vi "Hg-system-wendy.vi"() -> ()   [LabVIEW 2015]
uses:
  labview_Hg/XPALTC V 1.0 Andrey/Devices/Sirah Control 3 (provided by Sirah)/Addon/LabVIEW - Grobi API/Source/Laser/SC API Unit.ctl
panel:
  in  "VISA resource -Energy Meter 2":refnum<visa-resource-name>
  out "Current Pulse Energy Value 2":dbl=5.0 caption="Value"
  out "Current Pulse Energy Value Chart 2":dbl(graph)
  in  "VISA resource -Energy Meter":refnum<visa-resource-name>
  out "Current Pulse Energy Value":dbl=5.0 caption="Value"
  out "Current Pulse Energy Value Chart":dbl(graph)
  out "Current loop #":dbl format="%.4f"
  in  "# of Waveforms":i32
  in  "stop for waveform loop":bool
  out "Waveform Graph":dbl[](graph)
  in  "Channel":i32
  in  "VISA resource - Oscilliscope":refnum<visa-resource-name>
  out "Current Wavelength Read (nm)":dbl format="%.4f"
  out "Current Wavelength  Minus (nm)":dbl format="%.4f"
  in  "Boolean":bool
  out "Begin Wavelength Read (nm)":dbl format="%.4f"
  out "Begin Wavelength Read after laser go to (nm)":dbl format="%.4f"
  in  "Scan Step, nm":dbl
  in  "Scan to(longer), nm":dbl
  in  "Scan from (shorter), nm":dbl
  in  "VISA Resource - Dye Laser":refnum<visa-resource-name>
  out "error out":errorcluster
  in  "error in (no error)":errorcluster
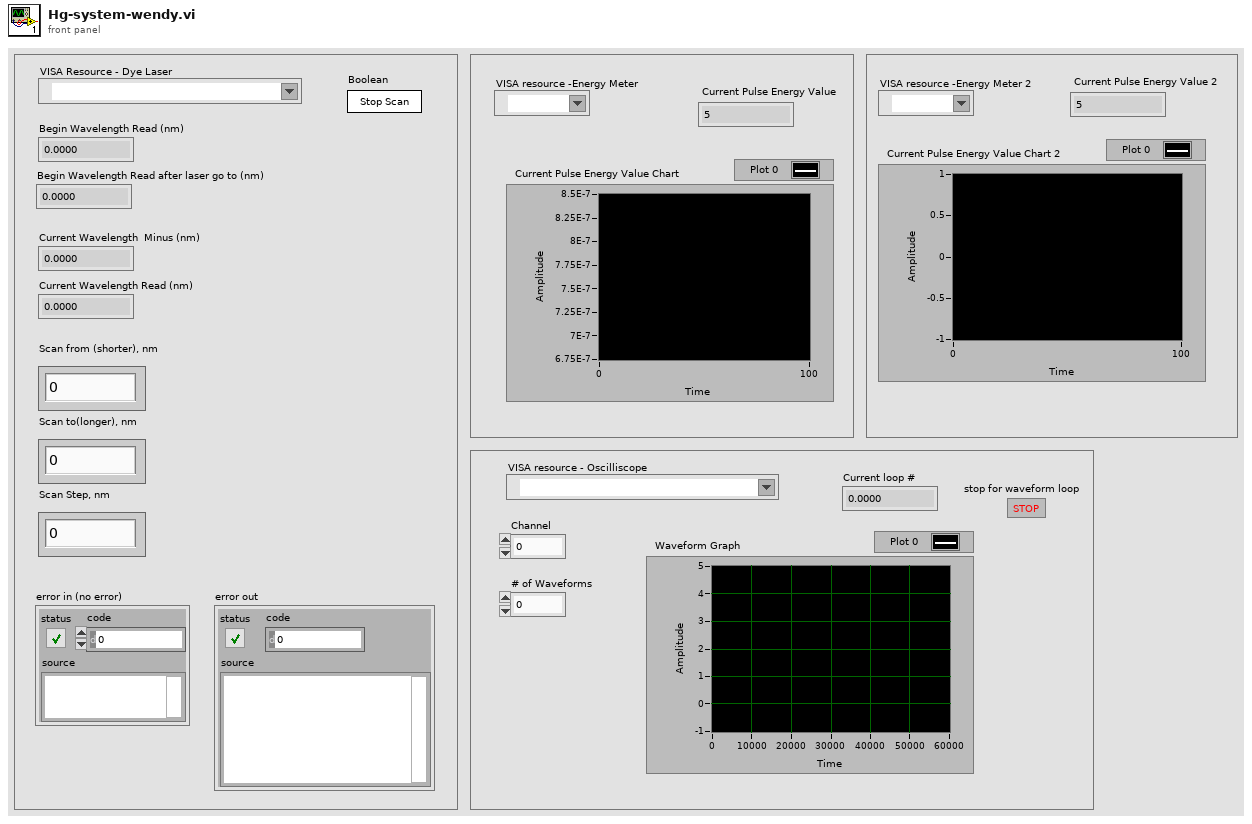
[diagram p1: front panel]
types:
  T1 = typedef "SC API Unit.ctl" = enum16{"nm", "THz", "1/cm"}
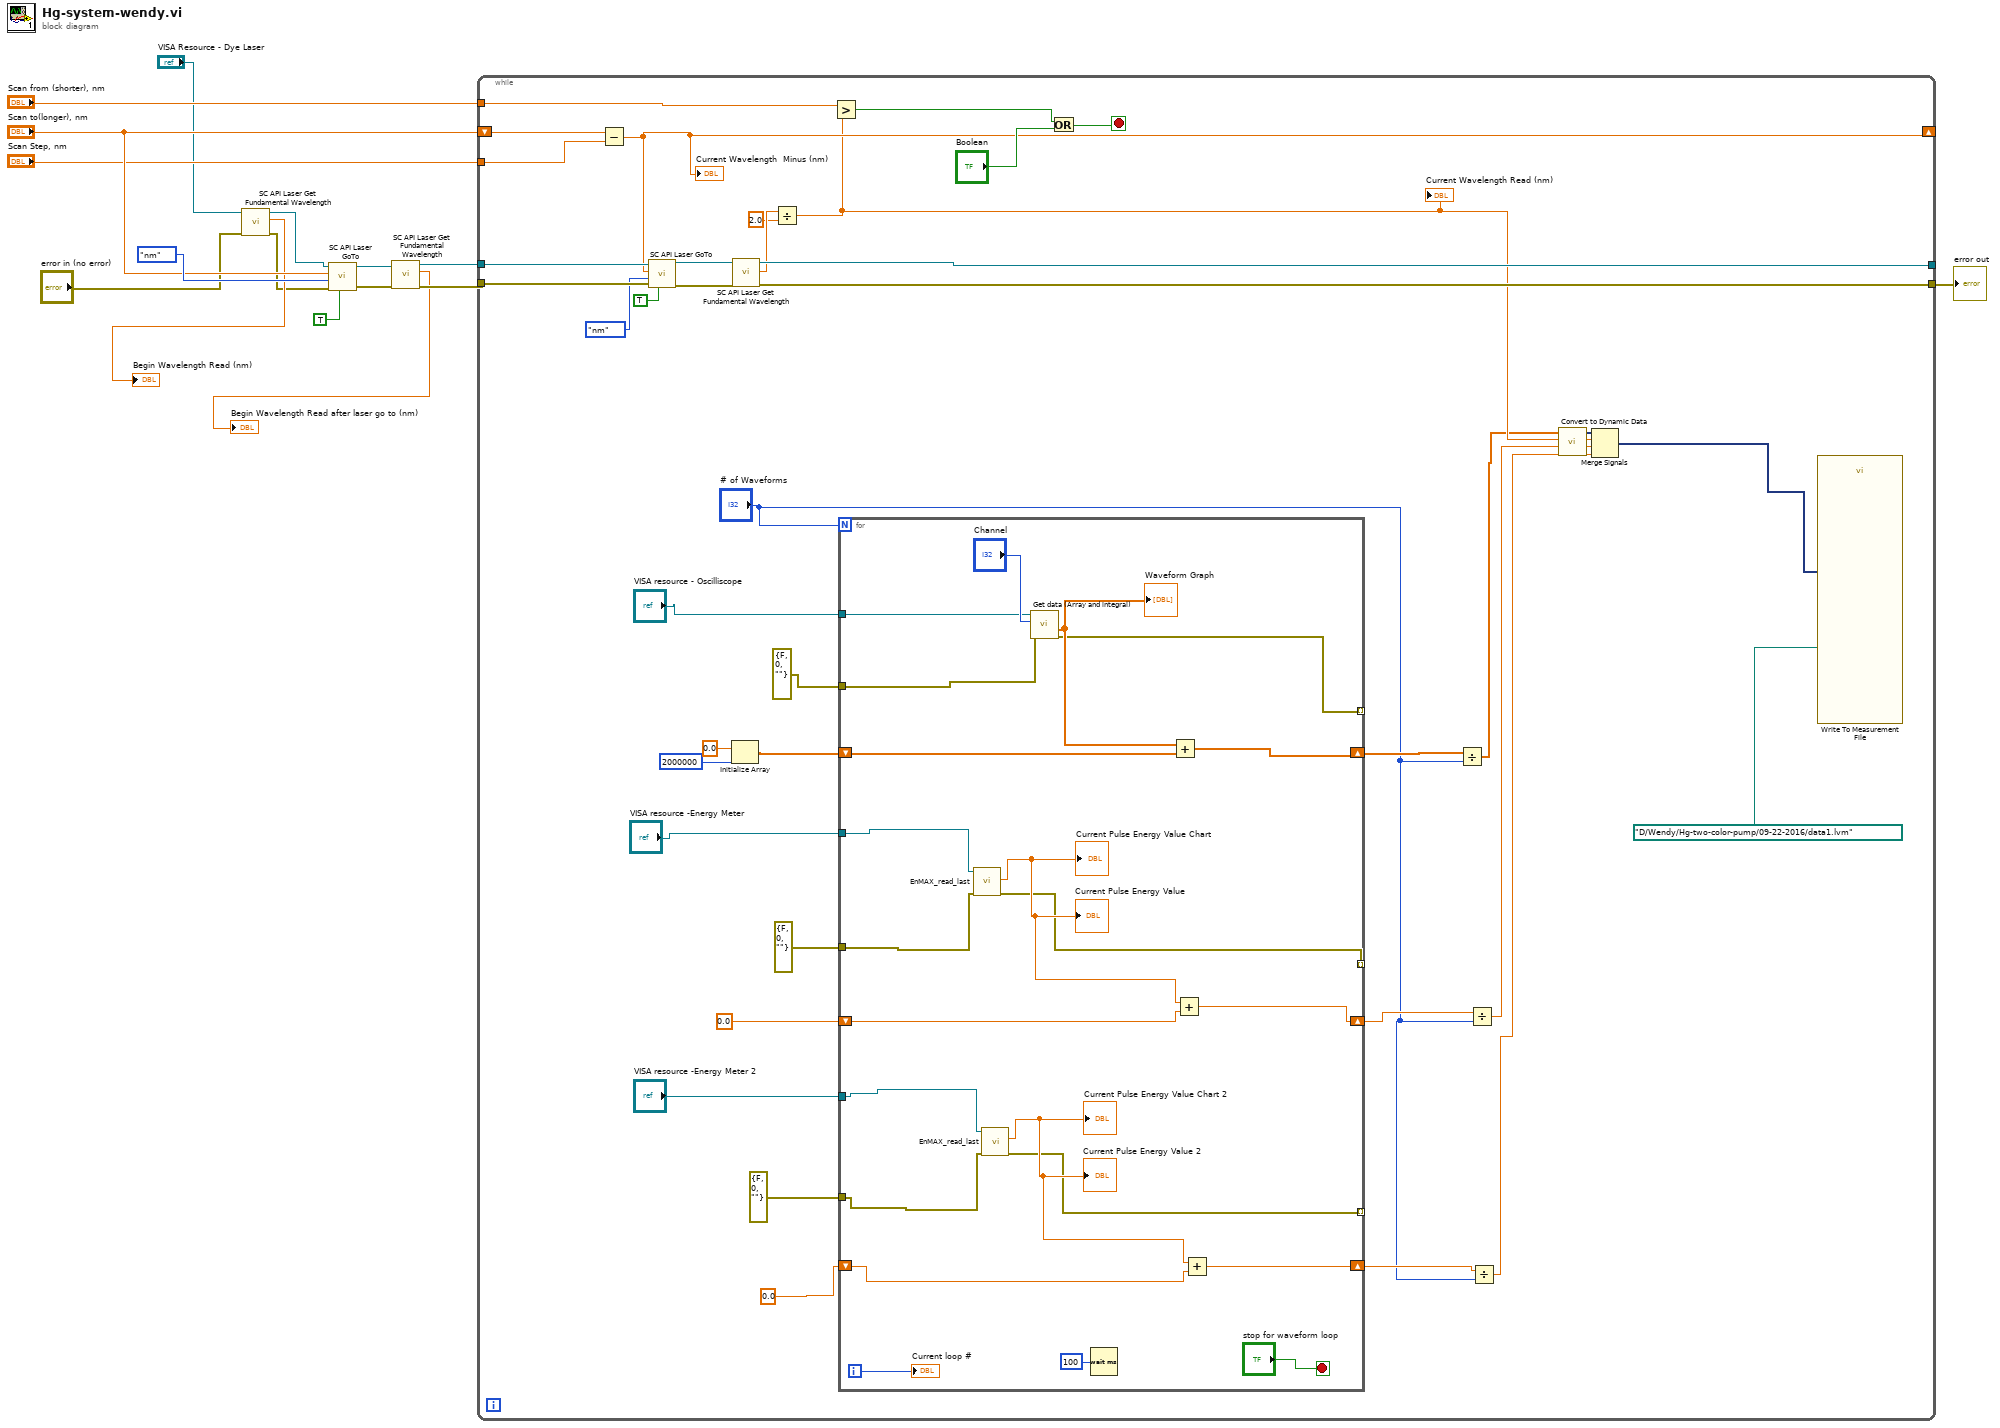
[diagram p0: block diagram]
diagram:
  n1 = call "SC API Laser Get Fundamental Wavelength.vi"("error in (no error)"="error in (no error)", "VISA Resource Name"="VISA Resource - Dye Laser") -> ("error out"=w1:errorcluster, "Current Wavelength (nm)"=→"Begin Wavelength Read (nm)":dbl, "VISA Resource Name Out"=w4:refnum<visa-resource-name>)  [unwired: 6 in, 1 out]
  n2 = call "SC API Laser GoTo.vi"("Wait for Completion? (FALSE)"=TRUE, "error in (no error)"=w1, "Unit"=SC_API_Unit."nm", "Wavelength (nm)"="Scan to(longer), nm", "VISA Resource Name"=w4) -> ("error out"=w13:errorcluster, "VISA Resource Name Out"=w16:refnum<visa-resource-name>)  [unwired: 5 in]
  n3 = call "SC API Laser Get Fundamental Wavelength.vi"("error in (no error)"=w13, "VISA Resource Name"=w16) -> ("error out"=w14:errorcluster, "Current Wavelength (nm)"=→"Begin Wavelength Read after laser go to (nm)":dbl, "VISA Resource Name Out"=w15:refnum<visa-resource-name>)  [unwired: 6 in, 1 out]
  n4 = while {
    tunnel: [w54] -> w10
    tunnel: [w53] -> _
    tunnel: w15 -> [w51]
    tunnel: w14 -> [w49]
    shift-right: [w28] -> _
    shift-left: "Scan to(longer), nm" -> [w48]
    tunnel: "Scan Step, nm" -> [w47]
    tunnel: "Scan from (shorter), nm" -> [w46]
    stop <- w42 stop-if-true
    n5 = Subtract(x=w48, y=w47) -> (x-y=w28:dbl)
    "Current Wavelength  Minus (nm)" <- w28
    n6 = call "SC API Laser GoTo.vi"("Wait for Completion? (FALSE)"=TRUE, "error in (no error)"=w49, "Unit"=SC_API_Unit."nm", "Wavelength (nm)"=w28, "VISA Resource Name"=w51) -> ("error out"=w55:errorcluster, "VISA Resource Name Out"=w52:refnum<visa-resource-name>)  [unwired: 5 in]
    n7 = Initialize Array(0.0 ("element"), 2000000 ("dimension size")) -> (w37:dbl[])
    n8 = call "SC API Laser Get Fundamental Wavelength.vi"("error in (no error)"=w55, "VISA Resource Name"=w52) -> ("error out"=w54:errorcluster, "Current Wavelength (nm)"=w41:dbl, "VISA Resource Name Out"=w53:refnum<visa-resource-name>)  [unwired: 6 in, 1 out]
    n9 = Divide(x=w41, y=2.0) -> (x/y=w27:dbl)
    "Current Wavelength Read (nm)" <- w27
    n10 = Greater?(x=w46, y=w27) -> (0:w43:bool)
    n11 = for {
      N: "# of Waveforms" -> [_]
      shift-right: [w73] -> w36
      shift-left: w37 -> [w74]
      tunnel: "VISA resource - Oscilliscope" -> [w70]
      tunnel: "VISA resource -Energy Meter" -> [w69]
      tunnel: errorcluster {"status"=FALSE, "code"=0, "source"=""} ("error in (no error)") -> [w68]
      tunnel: errorcluster {"status"=FALSE, "code"=0, "source"=""} ("error in (no error)") -> [w67]
      shift-right: [w64] -> w30
      shift-left: 0.0 ("y") -> [w65]
      tunnel: [w63] -> _ mode=indexing
      tunnel: [w62] -> _ mode=indexing
      tunnel: "VISA resource -Energy Meter 2" -> [w60]
      tunnel: errorcluster {"status"=FALSE, "code"=0, "source"=""} ("error in (no error)") -> [w59]
      tunnel: [w58] -> _ mode=indexing
      shift-right: [w57] -> w21
      shift-left: 0.0 ("y") -> [w56]
      i -> [w75]
      stop <- "stop for waveform loop" stop-if-true
      n12 = call "EnMAX_read_last.vi"("error in"=w67, "VISA in"=w69) -> ("error out"=w62:errorcluster, "Value"=w66:dbl)  [unwired: 7 in, 1 out]
      "Current Pulse Energy Value Chart" <- w66
      "Current Pulse Energy Value" <- w66
      n13 = call "EnMAX_read_last.vi"("error in"=w59, "VISA in"=w60) -> ("error out"=w58:errorcluster, "Value"=w61:dbl)  [unwired: 7 in, 1 out]
      "Current Pulse Energy Value Chart 2" <- w61
      "Current Pulse Energy Value 2" <- w61
      n14 = call "Get data (Array and integral).vi"("error in (no error)"=w68, "Channel"="Channel", "VISA resource name"=w70) -> ("error out"=w63:errorcluster, "array"=w72:dbl[])  [unwired: 6 in, 1 out]
      "Waveform Graph" <- w72
      n15 = Wait (ms)(milliseconds to wait=u32 100) -> ()  [unwired: 1 out]
      n16 = Add(x=w72, y=w74) -> (x+y=w73:dbl[])
      n17 = Add(x=w66, y=w65) -> (x+y=w64:dbl)
      n18 = Add(x=w61, y=w56) -> (x+y=w57:dbl)
      "Current loop #" <- w75
    }
    n19 = Or(x=w43, y="Boolean") -> (x .or. y?=w42:bool)
    n20 = Divide(x=w36, y="# of Waveforms") -> (x/y=w18:dbl[])
    n21 = Divide(x=w30, y="# of Waveforms") -> (x/y=w26:dbl)
    n22 = Divide(x=w21, y="# of Waveforms") -> (x/y=w19:dbl)
    n23 = call "Convert to Dynamic Data"("Array"=w18) -> ("Dynamic Data Type"=w17:dynamicdata)  [unwired: 3 in]
    n24 = Merge Signals(w17, w27, w26, w19) -> (w25:dynamicdata)
    n25 = call "Write To Measurement File"("Signals"=w25, "Filename"=path "D:/Wendy/Hg-two-color-pump/09-22-2016/data1.lvm") -> ()  [unwired: 15 in, 3 out]
  }
  "error out" <- w10
